vi "GT Set Rtc Time.vi"(8 "error in (no error)":errorcluster caption="错误输入（无错误）", 10 "pRtcTime":T1, 11 "cardNum":i16) -> (0 "error out":errorcluster caption="错误输出", 2 "pRtcTime out":T1, 3 "function return":i16)   [LabVIEW 2020, in "gts1.lvlib"]
doc: "GT_API GT_SetRtcTime(short cardNum,TRtcTime *pRtcTime);"
uses:
  gts1.lvlib
  dll/32bit/multi_card/gts.dll
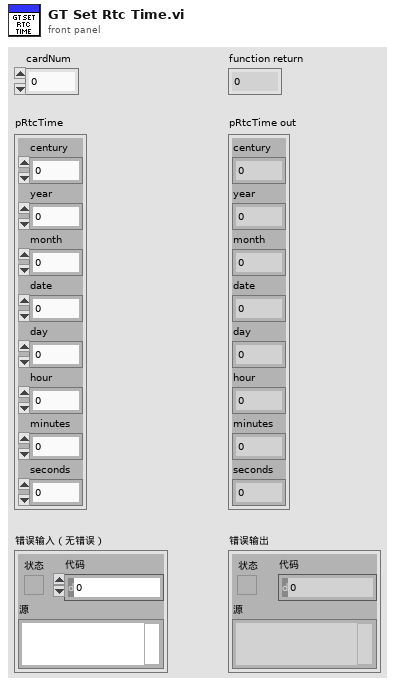
[diagram p1: front panel]
types:
  T1 = cluster{"century":i16, "year":i16, "month":i16, "date":i16, "day":i16, "hour":i16, "minutes":i16, "seconds":i16}
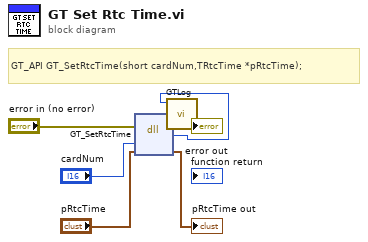
[diagram p0: block diagram]
diagram:
  # "GT_API GT_SetRtcTime(short cardNum,TRtcTime *pRtcTime);"
  n1 = dll-call lib="C:/1228/dll/32bit/multi_card/gts.dll" fn="GT_SetRtcTime"(error in="error in (no error)", "cardNum"="cardNum", "pRtcTime"="pRtcTime") -> (error out=w3:errorcluster, w1:i16, "pRtcTime"=→"pRtcTime out":T1)  [unwired: 3 in, 1 out]
  n2 = call "GTLog.vi"("error in (no error)"=w3, "Numeric"=w1) -> ("error out"=→"error out":errorcluster)  [unwired: 9 in]
